vi "Load by Name.vi"(8 "error in (no error)":errorcluster, 10 "Name":string, 11 "Plugin in":refnum<class "Plugin.lvclass">) -> (0 "error out":errorcluster, 3 "Plugin out":refnum<class "Plugin.lvclass">)   [LabVIEW 2018, in "neg-pkg.lvlib" / "Plugin.lvclass"]
uses:
  Plugin.lvclass
  <vilib>/regexp/Match Regular Expression.xnode
  neg-pkg.lvlib
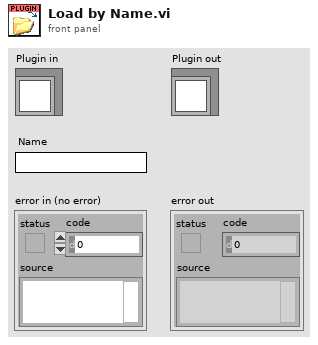
[diagram p1: front panel]
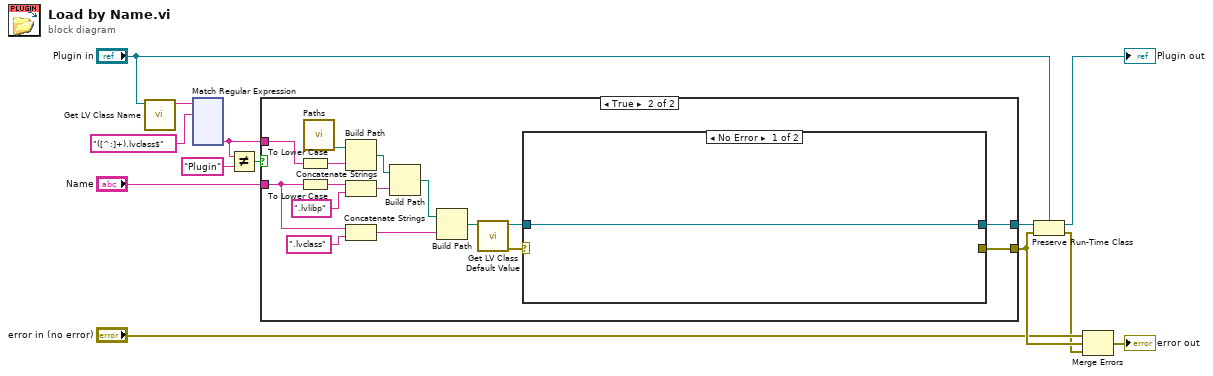
[diagram p0: block diagram]
diagram:
  n1 = call <vilib>:"Get LV Class Name.vi"("object"="Plugin in") -> ("class name"=w13:string)  [unwired: 9 in, 1 out]
  n2 = xnode "Match Regular Expression"("input string"=w13, "regular expression"="([^:]+).lvclass$") -> ("submatch 1"=w9:string)  [unwired: 4 in, 5 out]
  n3 = Not Equal?(x=w9, y="Plugin") -> (x != y?=w10:bool)
  n4 = case shown="True" w10 {
    tunnel: w9 -> [_ w29]
    tunnel: "Name" -> [_ w21]
    tunnel: [_ w15] -> w7
    tunnel: [_ w14] -> w3
    frame False {
    }
    frame True {
      n5 = To Lower Case(string=w29) -> (all lower case string=w24:string)
      n6 = To Lower Case(string=w21) -> (all lower case string=w23:string)
      n7 = call "Paths.vi"() -> ("ppl Path"=w28:path)  [unwired: 9 in, 2 out]
      n8 = Build Path(base path=w28, name or relative path=w24) -> (appended path=w27:path)
      n9 = Concatenate Strings(w23, ".lvlibp" ("string")) -> (w25:string)
      n10 = Concatenate Strings(w21, ".lvclass" ("string")) -> (w19:string)
      n11 = Build Path(base path=w27, name or relative path=w25) -> (appended path=w20:path)
      n12 = Build Path(base path=w20, name or relative path=w19) -> (appended path=w18:path)
      n13 = call <vilib>:"Get LV Class Default Value.vi"("class path"=w18) -> ("error out"=w17:errorcluster, "object"=w16:refnum<class>)  [unwired: 9 in]
      n14 = case shown="No Error" w17 {
        selector: w17 -> [_ w31]
        tunnel: w16 -> [w30 _]
        tunnel: [w30 _] -> w15
        tunnel: [_ w31] -> w14
        frame No Error {
        }
        frame Error {
        }
      }
    }
  }
  n15 = Preserve Run-Time Class(object in=w7, error in=w3, 2:"Plugin in") -> (object out=→"Plugin out":refnum<class "Plugin.lvclass">, error out=w1:errorcluster)
  n16 = Merge Errors("error in (no error)", w3, w1) -> (→"error out":errorcluster)
